vi "Test - Draw Teapot.vi"() -> ()   [LabVIEW 2022 SP3, in "Raster.lvlib"] (continued)
"UV"={"u"=0.0, "v"=0.0}, "Colour"=12517256}, "Vertex 2"={"Position"={"x"=671.18396, "y"=239.12437, "z"=0.9894685}, "UV"={"u"=0.0, "v"=0.0}, "Colour"=12517256}, "Vertex 3"={"Position"={"x"=666.5512, "y"=236.05386, "z"=0.9897306}, "UV"={"u"=0.0, "v"=0.0}, "Colour"=12517256}, "Alpha"=0.0, "Alpha Blending Enabled"=FALSE, "Colour"=131841}, {"Vertex 1"={"Position"={"x"=447.1671, "y"=407.3197, "z"=0.98938274}, "UV"={"u"=0.0, "v"=0.0}, "Colour"=12517256}, "Vertex 2"={"Position"={"x"=434.50436, "y"=408.5937, "z"=0.9895617}, "UV"={"u"=0.0, "v"=0.0}, "Colour"=12517256}, "Vertex 3"={"Position"={"x"=437.53577, "y"=407.4392, "z"=0.98967314}, "UV"={"u"=0.0, "v"=0.0}, "Colour"=12517256}, "Alpha"=0.0, "Alpha Blending Enabled"=FALSE, "Colour"=9618536}, {"Vertex 1"={"Position"={"x"=421.20996, "y"=448.31607, "z"=0.98949325}, "UV"={"u"=0.0, "v"=0.0}, "Colour"=12517256}, "Vertex 2"={"Position"={"x"=417.69724, "y"=440.7109, "z"=0.9895852}, "UV"={"u"=0.0, "v"=0.0}, "Colour"=12517256}, "Vertex 3"={"Position"={"x"=413.86533, "y"=441.3613, "z"=0.9895369}, "UV"={"u"=0.0, "v"=0.0}, "Colour"=12517256}, "Alpha"=0.0, "Alpha Blending Enabled"=FALSE, "Colour"=131841}, {"Vertex 1"={"Position"={"x"=400.0, "y"=130.68715, "z"=0.990049}, "UV"={"u"=0.0, "v"=0.0}, "Colour"=12517256}, "Vertex 2"={"Position"={"x"=413.89853, "y"=117.449425, "z"=0.9892527}, "UV"={"u"=0.0, "v"=0.0}, "Colour"=12517256}, "Vertex 3"={"Position"={"x"=420.06744, "y"=118.36189, "z"=0.9893066}, "UV"={"u"=0.0, "v"=0.0}, "Colour"=12517256}, "Alpha"=0.0, "Alpha Blending Enabled"=FALSE, "Colour"=131841}, {"Vertex 1"={"Position"={"x"=400.0, "y"=130.68715, "z"=0.990049}, "UV"={"u"=0.0, "v"=0.0}, "Colour"=12517256}, "Vertex 2"={"Position"={"x"=379.93253, "y"=118.36189, "z"=0.9893066}, "UV"={"u"=0.0, "v"=0.0}, "Colour"=12517256}, "Vertex 3"={"Position"={"x"=386.10147, "y"=117.449425, "z"=0.9892527}, "UV"={"u"=0.0, "v"=0.0}, "Colour"=12517256}, "Alpha"=0.0, "Alpha Blending Enabled"=FALSE, "Colour"=131841}, {"Vertex 1"={"Position"={"x"=437.2447, "y"=124.60762, "z"=0.98967606}, "UV"={"u"=0.0, "v"=0.0}, "Colour"=12517256}, "Vertex 2"={"Position"={"x"=469.5572, "y"=119.82906, "z"=0.98935246}, "UV"={"u"=0.0, "v"=0.0}, "Colour"=12517256}, "Vertex 3"={"Position"={"x"=472.6678, "y"=123.64719, "z"=0.9895792}, "UV"={"u"=0.0, "v"=0.0}, "Colour"=12517256}, "Alpha"=0.0, "Alpha Blending Enabled"=FALSE, "Colour"=131841}, {"Vertex 1"={"Position"={"x"=406.89297, "y"=415.6739, "z"=0.98965406}, "UV"={"u"=0.0, "v"=0.0}, "Colour"=12517256}, "Vertex 2"={"Position"={"x"=409.7829, "y"=413.03857, "z"=0.9894885}, "UV"={"u"=0.0, "v"=0.0}, "Colour"=12517256}, "Vertex 3"={"Position"={"x"=405.04242, "y"=413.28833, "z"=0.9894651}, "UV"={"u"=0.0, "v"=0.0}, "Colour"=12517256}, "Alpha"=0.0, "Alpha Blending Enabled"=FALSE, "Colour"=11792768}, {"Vertex 1"={"Position"={"x"=271.31854, "y"=391.44998, "z"=0.9896373}, "UV"={"u"=0.0, "v"=0.0}, "Colour"=12517256}, "Vertex 2"={"Position"={"x"=282.90906, "y"=394.1647, "z"=0.98967445}, "UV"={"u"=0.0, "v"=0.0}, "Colour"=12517256}, "Vertex 3"={"Position"={"x"=283.20917, "y"=397.61792, "z"=0.98929393}, "UV"={"u"=0.0, "v"=0.0}, "Colour"=12517256}, "Alpha"=0.0, "Alpha Blending Enabled"=FALSE, "Colour"=9091427}, {"Vertex 1"={"Position"={"x"=314.0461, "y"=401.00818, "z"=0.9894933}, "UV"={"u"=0.0, "v"=0.0}, "Colour"=12517256}, "Vertex 2"={"Position"={"x"=297.89752, "y"=399.48126, "z"=0.9893889}, "UV"={"u"=0.0, "v"=0.0}, "Colour"=12517256}, "Vertex 3"={"Position"={"x"=297.17767, "y"=396.39102, "z"=0.98972005}, "UV"={"u"=0.0, "v"=0.0}, "Colour"=12517256}, "Alpha"=0.0, "Alpha Blending Enabled"=FALSE, "Colour"=9091426}, {"Vertex 1"={"Position"={"x"=469.5572, "y"=119.82906, "z"=0.98935246}, "UV"={"u"=0.0, "v"=0.0}, "Colour"=12517256}, "Vertex 2"={"Position"={"x"=437.2447, "y"=124.60762, "z"=0.98967606}, "UV"={"u"=0.0, "v"=0.0}, "Colour"=12517256}, "Vertex 3"={"Position"={"x"=434.23392, "y"=122.73771, "z"=0.98956543}, "UV"={"u"=0.0, "v"=0.0}, "Colour"=12517256}, "Alpha"=0.0, "Alpha Blending Enabled"=FALSE, "Colour"=131841}, {"Vertex 1"={"Position"={"x"=437.53577, "y"=407.4392, "z"=0.98967314}, "UV"={"u"=0.0, "v"=0.0}, "Colour"=12517256}, "Vertex 2"={"Position"={"x"=451.1117, "y"=405.76608, "z"=0.98953724}, "UV"={"u"=0.0, "v"=0.0}, "Colour"=12517256}, "Vertex 3"={"Position"={"x"=447.1671, "y"=407.3197, "z"=0.98938274}, "UV"={"u"=0.0, "v"=0.0}, "Colour"=12517256}, "Alpha"=0.0, "Alpha Blending Enabled"=FALSE, "Colour"=9618536}, {"Vertex 1"={"Position"={"x"=392.3791, "y"=433.84442, "z"=0.9896132}, "UV"={"u"=0.0, "v"=0.0}, "Colour"=12517256}, "Vertex 2"={"Position"={"x"=390.40692, "y"=441.8486, "z"=0.98950064}, "UV"={"u"=0.0, "v"=0.0}, "Colour"=12517256}, "Vertex 3"={"Position"={"x"=395.05292, "y"=442.15393, "z"=0.98947793}, "UV"={"u"=0.0, "v"=0.0}, "Colour"=12517256}, "Alpha"=0.0, "Alpha Blending Enabled"=FALSE, "Colour"=461317}, {"Vertex 1"={"Position"={"x"=648.9251, "y"=288.04398, "z"=0.9894685}, "UV"={"u"=0.0, "v"=0.0}, "Colour"=12517256}, "Vertex 2"={"Position"={"x"=635.5962, "y"=277.87793, "z"=0.989419}, "UV"={"u"=0.0, "v"=0.0}, "Colour"=12517256}, "Vertex 3"={"Position"={"x"=627.5902, "y"=283.8639, "z"=0.98970413}, "UV"={"u"=0.0, "v"=0.0}, "Colour"=12517256}, "Alpha"=0.0, "Alpha Blending Enabled"=FALSE, "Colour"=10211695}, {"Vertex 1"={"Position"={"x"=396.44946, "y"=415.85388, "z"=0.98963785}, "UV"={"u"=0.0, "v"=0.0}, "Colour"=12517256}, "Vertex 2"={"Position"={"x"=394.9576, "y"=413.28833, "z"=0.9894651}, "UV"={"u"=0.0, "v"=0.0}, "Colour"=12517256}, "Vertex 3"={"Position"={"x"=390.2171, "y"=413.03857, "z"=0.9894885}, "UV"={"u"=0.0, "v"=0.0}, "Colour"=12517256}, "Alpha"=0.0, "Alpha Blending Enabled"=FALSE, "Colour"=11792768}, {"Vertex 1"={"Position"={"x"=690.8386, "y"=314.41168, "z"=0.98944694}, "UV"={"u"=0.0, "v"=0.0}, "Colour"=12517256}, "Vertex 2"={"Position"={"x"=695.06805, "y"=334.79984, "z"=0.98953646}, "UV"={"u"=0.0, "v"=0.0}, "Colour"=12517256}, "Vertex 3"={"Position"={"x"=698.27435, "y"=332.08707, "z"=0.9896034}, "UV"={"u"=0.0, "v"=0.0}, "Colour"=12517256}, "Alpha"=0.0, "Alpha Blending Enabled"=FALSE, "Colour"=7444305}, {"Vertex 1"={"Position"={"x"=425.77792, "y"=410.54718, "z"=0.98937297}, "UV"={"u"=0.0, "v"=0.0}, "Colour"=12517256}, "Vertex 2"={"Position"={"x"=418.06192, "y"=412.10922, "z"=0.98957527}, "UV"={"u"=0.0, "v"=0.0}, "Colour"=12517256}, "Vertex 3"={"Position"={"x"=421.46735, "y"=411.46152, "z"=0.9896358}, "UV"={"u"=0.0, "v"=0.0}, "Colour"=12517256}, "Alpha"=0.0, "Alpha Blending Enabled"=FALSE, "Colour"=10409073}, {"Vertex 1"={"Position"={"x"=409.72174, "y"=462.79736, "z"=0.98969}, "UV"={"u"=0.0, "v"=0.0}, "Colour"=12517256}, "Vertex 2"={"Position"={"x"=415.7588, "y"=463.67755, "z"=0.98946714}, "UV"={"u"=0.0, "v"=0.0}, "Colour"=12517256}, "Vertex 3"={"Position"={"x"=410.90912, "y"=464.3185, "z"=0.98942566}, "UV"={"u"=0.0, "v"=0.0}, "Colour"=12517256}, "Alpha"=0.0, "Alpha Blending Enabled"=FALSE, "Colour"=10343280}, {"Vertex 1"={"Position"={"x"=698.27435, "y"=332.08707, "z"=0.9896034}, "UV"={"u"=0.0, "v"=0.0}, "Colour"=12517256}, "Vertex 2"={"Position"={"x"=693.37805, "y"=310.46698, "z"=0.98952615}, "UV"={"u"=0.0, "v"=0.0}, "Colour"=12517256}, "Vertex 3"={"Position"={"x"=690.8386, "y"=314.41168, "z"=0.98944694}, "UV"={"u"=0.0, "v"=0.0}, "Colour"=12517256}, "Alpha"=0.0, "Alpha Blending Enabled"=FALSE, "Colour"=6522183}, {"Vertex 1"={"Position"={"x"=403.92798, "y"=434.0735, "z"=0.9895953}, "UV"={"u"=0.0, "v"=0.0}, "Colour"=12517256}, "Vertex 2"={"Position"={"x"=404.94708, "y"=442.15393, "z"=0.98947793}, "UV"={"u"=0.0, "v"=0.0}, "Colour"=12517256}, "Vertex 3"={"Position"={"x"=409.59305, "y"=441.8486, "z"=0.98950064}, "UV"={"u"=0.0, "v"=0.0}, "Colour"=12517256}, "Alpha"=0.0, "Alpha Blending Enabled"=FALSE, "Colour"=461317}, {"Vertex 1"={"Position"={"x"=427.9001, "y"=453.91602, "z"=0.98951197}, "UV"={"u"=0.0, "v"=0.0}, "Colour"=12517256}, "Vertex 2"={"Position"={"x"=425.17258, "y"=447.3146, "z"=0.98956454}, "UV"={"u"=0.0, "v"=0.0}, "Colour"=12517256}, "Vertex 3"={"Position"={"x"=421.20996, "y"=448.31607, "z"=0.98949325}, "UV"={"u"=0.0, "v"=0.0}, "Colour"=12517256}, "Alpha"=0.0, "Alpha Blending Enabled"=FALSE, "Colour"=988427}, {"Vertex 1"={"Position"={"x"=657.4915, "y"=300.53033, "z"=0.9895282}, "UV"={"u"=0.0, "v"=0.0}, "Colour"=12517256}, "Vertex 2"={"Position"={"x"=662.8395, "y"=314.53314, "z"=0.9895922}, "UV"={"u"=0.0, "v"=0.0}, "Colour"=12517256}, "Vertex 3"={"Position"={"x"=670.3497, "y"=310.34482, "z"=0.9894408}, "UV"={"u"=0.0, "v"=0.0}, "Colour"=12517256}, "Alpha"=0.0, "Alpha Blending Enabled"=FALSE, "Colour"=9354853}, {"Vertex 1"={"Position"={"x"=403.55054, "y"=415.85388, "z"=0.98963785}, "UV"={"u"=0.0, "v"=0.0}, "Colour"=12517256}, "Vertex 2"={"Position"={"x"=405.04242, "y"=413.28833, "z"=0.9894651}, "UV"={"u"=0.0, "v"=0.0}, "Colour"=12517256}, "Vertex 3"={"Position"={"x"=400.0, "y"=413.3747, "z"=0.9894571}, "UV"={"u"=0.0, "v"=0.0}, "Colour"=12517256}, "Alpha"=0.0, "Alpha Blending Enabled"=FALSE, "Colour"=11924353}, {"Vertex 1"={"Position"={"x"=673.70026, "y"=326.4925, "z"=0.98952615}, "UV"={"u"=0.0, "v"=0.0}, "Colour"=12517256}, "Vertex 2"={"Position"={"x"=670.3497, "y"=310.34482, "z"=0.9894408}, "UV"={"u"=0.0, "v"=0.0}, "Colour"=12517256}, "Vertex 3"={"Position"={"x"=662.8395, "y"=314.53314, "z"=0.9895922}, "UV"={"u"=0.0, "v"=0.0}, "Colour"=12517256}, "Alpha"=0.0, "Alpha Blending Enabled"=FALSE, "Colour"=8630110}, {"Vertex 1"={"Position"={"x"=393.28003, "y"=463.19003, "z"=0.98966503}, "UV"={"u"=0.0, "v"=0.0}, "Colour"=12517256}, "Vertex 2"={"Position"={"x"=389.09088, "y"=464.3185, "z"=0.98942566}, "UV"={"u"=0.0, "v"=0.0}, "Colour"=12517256}, "Vertex 3"={"Position"={"x"=384.2412, "y"=463.67755, "z"=0.98946714}, "UV"={"u"=0.0, "v"=0.0}, "Colour"=12517256}, "Alpha"=0.0, "Alpha Blending Enabled"=FALSE, "Colour"=10343280}, {"Vertex 1"={"Position"={"x"=383.36658, "y"=449.1381, "z"=0.9894347}, "UV"={"u"=0.0, "v"=0.0}, "Colour"=12517256}, "Vertex 2"={"Position"={"x"=386.13464, "y"=441.3613, "z"=0.9895369}, "UV"={"u"=0.0, "v"=0.0}, "Colour"=12517256}, "Vertex 3"={"Position"={"x"=382.30276, "y"=440.7109, "z"=0.9895852}, "UV"={"u"=0.0, "v"=0.0}, "Colour"=12517256}, "Alpha"=0.0, "Alpha Blending Enabled"=FALSE, "Colour"=131841}, {"Vertex 1"={"Position"={"x"=400.0, "y"=415.91602, "z"=0.9896323}, "UV"={"u"=0.0, "v"=0.0}, "Colour"=12517256}, "Vertex 2"={"Position"={"x"=400.0, "y"=413.3747, "z"=0.9894571}, "UV"={"u"=0.0, "v"=0.0}, "Colour"=12517256}, "Vertex 3"={"Position"={"x"=394.9576, "y"=413.28833, "z"=0.9894651}, "UV"={"u"=0.0, "v"=0.0}, "Colour"=12517256}, "Alpha"=0.0, "Alpha Blending Enabled"=FALSE, "Colour"=11924353}, {"Vertex 1"={"Position"={"x"=423.5128, "y"=460.18484, "z"=0.98943293}, "UV"={"u"=0.0, "v"=0.0}, "Colour"=12517256}, "Vertex 2"={"Position"={"x"=420.0997, "y"=462.82288, "z"=0.98952234}, "UV"={"u"=0.0, "v"=0.0}, "Colour"=12517256}, "Vertex 3"={"Position"={"x"=423.8626, "y"=461.78098, "z"=0.98958975}, "UV"={"u"=0.0, "v"=0.0}, "Colour"=12517256}, "Alpha"=0.0, "Alpha Blending Enabled"=FALSE, "Colour"=11133561}, {"Vertex 1"={"Position"={"x"=396.07202, "y"=434.0735, "z"=0.9895953}, "UV"={"u"=0.0, "v"=0.0}, "Colour"=12517256}, "Vertex 2"={"Position"={"x"=395.05292, "y"=442.15393, "z"=0.98947793}, "UV"={"u"=0.0, "v"=0.0}, "Colour"=12517256}, "Vertex 3"={"Position"={"x"=400.0, "y"=442.25943, "z"=0.98947006}, "UV"={"u"=0.0, "v"=0.0}, "Colour"=12517256}, "Alpha"=0.0, "Alpha Blending Enabled"=FALSE, "Colour"=658951}, {"Vertex 1"={"Position"={"x"=400.0, "y"=434.1526, "z"=0.9895892}, "UV"={"u"=0.0, "v"=0.0}, "Colour"=12517256}, "Vertex 2"={"Position"={"x"=400.0, "y"=442.25943, "z"=0.98947006}, "UV"={"u"=0.0, "v"=0.0}, "Colour"=12517256}, "Vertex 3"={"Position"={"x"=404.94708, "y"=442.15393, "z"=0.98947793}, "UV"={"u"=0.0, "v"=0.0}, "Colour"=12517256}, "Alpha"=0.0, "Alpha Blending Enabled"=FALSE, "Colour"=658951}, {"Vertex 1"={"Position"={"x"=423.8626, "y"=461.78098, "z"=0.98958975}, "UV"={"u"=0.0, "v"=0.0}, "Colour"=12517256}, "Vertex 2"={"Position"={"x"=427.8845, "y"=458.98697, "z"=0.9895123}, "UV"={"u"=0.0, "v"=0.0}, "Colour"=12517256}, "Vertex 3"={"Position"={"x"=423.5128, "y"=460.18484, "z"=0.98943293}, "UV"={"u"=0.0, "v"=0.0}, "Colour"=12517256}, "Alpha"=0.0, "Alpha Blending Enabled"=FALSE, "Colour"=11133561}, {"Vertex 1"={"Position"={"x"=537.5546, "y"=128.3227, "z"=0.989609}, "UV"={"u"=0.0, "v"=0.0}, "Colour"=12517256}, "Vertex 2"={"Position"={"x"=521.88995, "y"=127.45417, "z"=0.9896591}, "UV"={"u"=0.0, "v"=0.0}, "Colour"=12517256}, "Vertex 3"={"Position"={"x"=521.76056, "y"=120.85737, "z"=0.98926175}, "UV"={"u"=0.0, "v"=0.0}, "Colour"=12517256}, "Alpha"=0.0, "Alpha Blending Enabled"=FALSE, "Colour"=131841}, {"Vertex 1"={"Position"={"x"=517.09094, "y"=394.1647, "z"=0.98967445}, "UV"={"u"=0.0, "v"=0.0}, "Colour"=12517256}, "Vertex 2"={"Position"={"x"=528.68146, "y"=391.44998, "z"=0.9896373}, "UV"={"u"=0.0, "v"=0.0}, "Colour"=12517256}, "Vertex 3"={"Position"={"x"=528.8192, "y"=395.14902, "z"=0.98921615}, "UV"={"u"=0.0, "v"=0.0}, "Colour"=12517256}, "Alpha"=0.0, "Alpha Blending Enabled"=FALSE, "Colour"=9091427}, {"Vertex 1"={"Position"={"x"=348.88834, "y"=405.76608, "z"=0.98953724}, "UV"={"u"=0.0, "v"=0.0}, "Colour"=12517256}, "Vertex 2"={"Position"={"x"=333.56543, "y"=404.58322, "z"=0.98938376}, "UV"={"u"=0.0, "v"=0.0}, "Colour"=12517256}, "Vertex 3"={"Position"={"x"=330.52844, "y"=402.4644, "z"=0.9895999}, "UV"={"u"=0.0, "v"=0.0}, "Colour"=12517256}, "Alpha"=0.0, "Alpha Blending Enabled"=FALSE, "Colour"=9289061}, {"Vertex 1"={"Position"={"x"=400.0, "y"=130.68715, "z"=0.990049}, "UV"={"u"=0.0, "v"=0.0}, "Colour"=12517256}, "Vertex 2"={"Position"={"x"=407.17038, "y"=116.87585, "z"=0.9892187}, "UV"={"u"=0.0, "v"=0.0}, "Colour"=12517256}, "Vertex 3"={"Position"={"x"=413.89853, "y"=117.449425, "z"=0.9892527}, "UV"={"u"=0.0, "v"=0.0}, "Colour"=12517256}, "Alpha"=0.0, "Alpha Blending Enabled"=FALSE, "Colour"=131841}, {"Vertex 1"={"Position"={"x"=400.0, "y"=130.68715, "z"=0.990049}, "UV"={"u"=0.0, "v"=0.0}, "Colour"=12517256}, "Vertex 2"={"Position"={"x"=386.10147, "y"=117.449425, "z"=0.9892527}, "UV"={"u"=0.0, "v"=0.0}, "Colour"=12517256}, "Vertex 3"={"Position"={"x"=392.82962, "y"=116.87585, "z"=0.9892187}, "UV"={"u"=0.0, "v"=0.0}, "Colour"=12517256}, "Alpha"=0.0, "Alpha Blending Enabled"=FALSE, "Colour"=131841}, {"Vertex 1"={"Position"={"x"=382.30276, "y"=440.7109, "z"=0.9895852}, "UV"={"u"=0.0, "v"=0.0}, "Colour"=12517256}, "Vertex 2"={"Position"={"x"=378.79004, "y"=448.31607, "z"=0.98949325}, "UV"={"u"=0.0, "v"=0.0}, "Colour"=12517256}, "Vertex 3"={"Position"={"x"=383.36658, "y"=449.1381, "z"=0.9894347}, "UV"={"u"=0.0, "v"=0.0}, "Colour"=12517256}, "Alpha"=0.0, "Alpha Blending Enabled"=FALSE, "Colour"=131841}, {"Vertex 1"={"Position"={"x"=683.931, "y"=340.25684, "z"=0.98953646}, "UV"={"u"=0.0, "v"=0.0}, "Colour"=12517256}, "Vertex 2"={"Position"={"x"=680.5069, "y"=322.8259, "z"=0.98944694}, "UV"={"u"=0.0, "v"=0.0}, "Colour"=12517256}, "Vertex 3"={"Position"={"x"=673.70026, "y"=326.4925, "z"=0.98952615}, "UV"={"u"=0.0, "v"=0.0}, "Colour"=12517256}, "Alpha"=0.0, "Alpha Blending Enabled"=FALSE, "Colour"=10540658}, {"Vertex 1"={"Position"={"x"=374.82742, "y"=447.3146, "z"=0.98956454}, "UV"={"u"=0.0, "v"=0.0}, "Colour"=12517256}, "Vertex 2"={"Position"={"x"=372.0999, "y"=453.91602, "z"=0.98951197}, "UV"={"u"=0.0, "v"=0.0}, "Colour"=12517256}, "Vertex 3"={"Position"={"x"=376.47418, "y"=455.0764, "z"=0.9894326}, "UV"={"u"=0.0, "v"=0.0}, "Colour"=12517256}, "Alpha"=0.0, "Alpha Blending Enabled"=FALSE, "Colour"=988427}, {"Vertex 1"={"Position"={"x"=626.93384, "y"=205.09799, "z"=0.989385}, "UV"={"u"=0.0, "v"=0.0}, "Colour"=12517256}, "Vertex 2"={"Position"={"x"=653.6545, "y"=220.1329, "z"=0.989419}, "UV"={"u"=0.0, "v"=0.0}, "Colour"=12517256}, "Vertex 3"={"Position"={"x"=648.53705, "y"=216.88268, "z"=0.98970413}, "UV"={"u"=0.0, "v"=0.0}, "Colour"=12517256}, "Alpha"=0.0, "Alpha Blending Enabled"=FALSE, "Colour"=131841}, {"Vertex 1"={"Position"={"x"=680.5069, "y"=322.8259, "z"=0.98944694}, "UV"={"u"=0.0, "v"=0.0}, "Colour"=12517256}, "Vertex 2"={"Position"={"x"=683.931, "y"=340.25684, "z"=0.98953646}, "UV"={"u"=0.0, "v"=0.0}, "Colour"=12517256}, "Vertex 3"={"Position"={"x"=690.1191, "y"=337.60867, "z"=0.98951393}, "UV"={"u"=0.0, "v"=0.0}, "Colour"=12517256}, "Alpha"=0.0, "Alpha Blending Enabled"=FALSE, "Colour"=10804598}, {"Vertex 1"={"Position"={"x"=376.47418, "y"=455.0764, "z"=0.9894326}, "UV"={"u"=0.0, "v"=0.0}, "Colour"=12517256}, "Vertex 2"={"Position"={"x"=378.79004, "y"=448.31607, "z"=0.98949325}, "UV"={"u"=0.0, "v"=0.0}, "Colour"=12517256}, "Vertex 3"={"Position"={"x"=374.82742, "y"=447.3146, "z"=0.98956454}, "UV"={"u"=0.0, "v"=0.0}, "Colour"=12517256}, "Alpha"=0.0, "Alpha Blending Enabled"=FALSE, "Colour"=988427}, {"Vertex 1"={"Position"={"x"=406.71997, "y"=463.19003, "z"=0.98966503}, "UV"={"u"=0.0, "v"=0.0}, "Colour"=12517256}, "Vertex 2"={"Position"={"x"=410.90912, "y"=464.3185, "z"=0.98942566}, "UV"={"u"=0.0, "v"=0.0}, "Colour"=12517256}, "Vertex 3"={"Position"={"x"=405.62814, "y"=464.7204, "z"=0.9893997}, "UV"={"u"=0.0, "v"=0.0}, "Colour"=12517256}, "Alpha"=0.0, "Alpha Blending Enabled"=FALSE, "Colour"=10409073}, {"Vertex 1"={"Position"={"x"=635.5962, "y"=277.87793, "z"=0.989419}, "UV"={"u"=0.0, "v"=0.0}, "Colour"=12517256}, "Vertex 2"={"Position"={"x"=615.98, "y"=270.86078, "z"=0.989385}, "UV"={"u"=0.0, "v"=0.0}, "Colour"=12517256}, "Vertex 3"={"Position"={"x"=608.8621, "y"=277.8157, "z"=0.9896861}, "UV"={"u"=0.0, "v"=0.0}, "Colour"=12517256}, "Alpha"=0.0, "Alpha Blending Enabled"=FALSE, "Colour"=11265402}, {"Vertex 1"={"Position"={"x"=365.49564, "y"=408.5937, "z"=0.9895617}, "UV"={"u"=0.0, "v"=0.0}, "Colour"=12517256}, "Vertex 2"={"Position"={"x"=352.83286, "y"=407.3197, "z"=0.98938274}, "UV"={"u"=0.0, "v"=0.0}, "Colour"=12517256}, "Vertex 3"={"Position"={"x"=348.88834, "y"=405.76608, "z"=0.98953724}, "UV"={"u"=0.0, "v"=0.0}, "Colour"=12517256}, "Alpha"=0.0, "Alpha Blending Enabled"=FALSE, "Colour"=9618536}, {"Vertex 1"={"Position"={"x"=314.0461, "y"=401.00818, "z"=0.9894933}, "UV"={"u"=0.0, "v"=0.0}, "Colour"=12517256}, "Vertex 2"={"Position"={"x"=330.52844, "y"=402.4644, "z"=0.9895999}, "UV"={"u"=0.0, "v"=0.0}, "Colour"=12517256}, "Vertex 3"={"Position"={"x"=333.56543, "y"=404.58322, "z"=0.98938376}, "UV"={"u"=0.0, "v"=0.0}, "Colour"=12517256}, "Alpha"=0.0, "Alpha Blending Enabled"=FALSE, "Colour"=9289061}, {"Vertex 1"={"Position"={"x"=400.0, "y"=130.68715, "z"=0.990049}, "UV"={"u"=0.0, "v"=0.0}, "Colour"=12517256}, "Vertex 2"={"Position"={"x"=400.0, "y"=116.67725, "z"=0.989207}, "UV"={"u"=0.0, "v"=0.0}, "Colour"=12517256}, "Vertex 3"={"Position"={"x"=407.17038, "y"=116.87585, "z"=0.9892187}, "UV"={"u"=0.0, "v"=0.0}, "Colour"=12517256}, "Alpha"=0.0, "Alpha Blending Enabled"=FALSE, "Colour"=131841}, {"Vertex 1"={"Position"={"x"=400.0, "y"=130.68715, "z"=0.990049}, "UV"={"u"=0.0, "v"=0.0}, "Colour"=12517256}, "Vertex 2"={"Position"={"x"=392.82962, "y"=116.87585, "z"=0.9892187}, "UV"={"u"=0.0, "v"=0.0}, "Colour"=12517256}, "Vertex 3"={"Position"={"x"=400.0, "y"=116.67725, "z"=0.989207}, "UV"={"u"=0.0, "v"=0.0}, "Colour"=12517256}, "Alpha"=0.0, "Alpha Blending Enabled"=FALSE, "Colour"=131841}, {"Vertex 1"={"Position"={"x"=396.5364, "y"=463.4357, "z"=0.9896494}, "UV"={"u"=0.0, "v"=0.0}, "Colour"=12517256}, "Vertex 2"={"Position"={"x"=394.37186, "y"=464.7204, "z"=0.9893997}, "UV"={"u"=0.0, "v"=0.0}, "Colour"=12517256}, "Vertex 3"={"Position"={"x"=389.09088, "y"=464.3185, "z"=0.98942566}, "UV"={"u"=0.0, "v"=0.0}, "Colour"=12517256}, "Alpha"=0.0, "Alpha Blending Enabled"=FALSE, "Colour"=10409073}, {"Vertex 1"={"Position"={"x"=688.6595, "y"=283.87192, "z"=0.9895922}, "UV"={"u"=0.0, "v"=0.0}, "Colour"=12517256}, "Vertex 2"={"Position"={"x"=682.01483, "y"=260.7837, "z"=0.9895282}, "UV"={"u"=0.0, "v"=0.0}, "Colour"=12517256}, "Vertex 3"={"Position"={"x"=683.1556, "y"=265.8486, "z"=0.9893541}, "UV"={"u"=0.0, "v"=0.0}, "Colour"=12517256}, "Alpha"=0.0, "Alpha Blending Enabled"=FALSE, "Colour"=2305817}, {"Vertex 1"={"Position"={"x"=374.2221, "y"=410.54718, "z"=0.98937297}, "UV"={"u"=0.0, "v"=0.0}, "Colour"=12517256}, "Vertex 2"={"Position"={"x"=381.9381, "y"=412.10922, "z"=0.98957527}, "UV"={"u"=0.0, "v"=0.0}, "Colour"=12517256}, "Vertex 3"={"Position"={"x"=385.85406, "y"=412.64026, "z"=0.98952574}, "UV"={"u"=0.0, "v"=0.0}, "Colour"=12517256}, "Alpha"=0.0, "Alpha Blending Enabled"=FALSE, "Colour"=10672500}, {"Vertex 1"={"Position"={"x"=416.63342, "y"=449.1381, "z"=0.9894347}, "UV"={"u"=0.0, "v"=0.0}, "Colour"=12517256}, "Vertex 2"={"Position"={"x"=413.86533, "y"=441.3613, "z"=0.9895369}, "UV"={"u"=0.0, "v"=0.0}, "Colour"=12517256}, "Vertex 3"={"Position"={"x"=409.59305, "y"=441.8486, "z"=0.98950064}, "UV"={"u"=0.0, "v"=0.0}, "Colour"=12517256}, "Alpha"=0.0, "Alpha Blending Enabled"=FALSE, "Colour"=263427}, {"Vertex 1"={"Position"={"x"=686.3912, "y"=318.6656, "z"=0.9894203}, "UV"={"u"=0.0, "v"=0.0}, "Colour"=12517256}, "Vertex 2"={"Position"={"x"=690.1191, "y"=337.60867, "z"=0.98951393}, "UV"={"u"=0.0, "v"=0.0}, "Colour"=12517256}, "Vertex 3"={"Position"={"x"=695.06805, "y"=334.79984, "z"=0.98953646}, "UV"={"u"=0.0, "v"=0.0}, "Colour"=12517256}, "Alpha"=0.0, "Alpha Blending Enabled"=FALSE, "Colour"=9750122}, {"Vertex 1"={"Position"={"x"=421.46735, "y"=411.46152, "z"=0.9896358}, "UV"={"u"=0.0, "v"=0.0}, "Colour"=12517256}, "Vertex 2"={"Position"={"x"=430.5626, "y"=409.63797, "z"=0.98946077}, "UV"={"u"=0.0, "v"=0.0}, "Colour"=12517256}, "Vertex 3"={"Position"={"x"=425.77792, "y"=410.54718, "z"=0.98937297}, "UV"={"u"=0.0, "v"=0.0}, "Colour"=12517256}, "Alpha"=0.0, "Alpha Blending Enabled"=FALSE, "Colour"=10409073}, {"Vertex 1"={"Position"={"x"=379.9003, "y"=462.82288, "z"=0.98952234}, "UV"={"u"=0.0, "v"=0.0}, "Colour"=12517256}, "Vertex 2"={"Position"={"x"=376.4872, "y"=460.18484, "z"=0.98943293}, "UV"={"u"=0.0, "v"=0.0}, "Colour"=12517256}, "Vertex 3"={"Position"={"x"=372.1155, "y"=458.98697, "z"=0.9895123}, "UV"={"u"=0.0, "v"=0.0}, "Colour"=12517256}, "Alpha"=0.0, "Alpha Blending Enabled"=FALSE, "Colour"=11133561}, {"Vertex 1"={"Position"={"x"=263.53796, "y"=388.02435, "z"=0.98961246}, "UV"={"u"=0.0, "v"=0.0}, "Colour"=12517256}, "Vertex 2"={"Position"={"x"=271.31854, "y"=391.44998, "z"=0.9896373}, "UV"={"u"=0.0, "v"=0.0}, "Colour"=12517256}, "Vertex 3"={"Position"={"x"=271.1808, "y"=395.14902, "z"=0.98921615}, "UV"={"u"=0.0, "v"=0.0}, "Colour"=12517256}, "Alpha"=0.0, "Alpha Blending Enabled"=FALSE, "Colour"=8893792}, {"Vertex 1"={"Position"={"x"=413.86533, "y"=441.3613, "z"=0.9895369}, "UV"={"u"=0.0, "v"=0.0}, "Colour"=12517256}, "Vertex 2"={"Position"={"x"=416.63342, "y"=449.1381, "z"=0.9894347}, "UV"={"u"=0.0, "v"=0.0}, "Colour"=12517256}, "Vertex 3"={"Position"={"x"=421.20996, "y"=448.31607, "z"=0.98949325}, "UV"={"u"=0.0, "v"=0.0}, "Colour"=12517256}, "Alpha"=0.0, "Alpha Blending Enabled"=FALSE, "Colour"=131841}, {"Vertex 1"={"Position"={"x"=372.0999, "y"=453.91602, "z"=0.98951197}, "UV"={"u"=0.0, "v"=0.0}, "Colour"=12517256}, "Vertex 2"={"Position"={"x"=372.1155, "y"=458.98697, "z"=0.9895123}, "UV"={"u"=0.0, "v"=0.0}, "Colour"=12517256}, "Vertex 3"={"Position"={"x"=376.4872, "y"=460.18484, "z"=0.98943293}, "UV"={"u"=0.0, "v"=0.0}, "Colour"=12517256}, "Alpha"=0.0, "Alpha Blending Enabled"=FALSE, "Colour"=6785610}, {"Vertex 1"={"Position"={"x"=427.8845, "y"=458.98697, "z"=0.9895123}, "UV"={"u"=0.0, "v"=0.0}, "Colour"=12517256}, "Vertex 2"={"Position"={"x"=427.9001, "y"=453.91602, "z"=0.98951197}, "UV"={"u"=0.0, "v"=0.0}, "Colour"=12517256}, "Vertex 3"={"Position"={"x"=423.52582, "y"=455.0764, "z"=0.9894326}, "UV"={"u"=0.0, "v"=0.0}, "Colour"=12517256}, "Alpha"=0.0, "Alpha Blending Enabled"=FALSE, "Colour"=6785610}, {"Vertex 1"={"Position"={"x"=588.6202, "y"=195.32538, "z"=0.9893725}, "UV"={"u"=0.0, "v"=0.0}, "Colour"=12517256}, "Vertex 2"={"Position"={"x"=626.93384, "y"=205.09799, "z"=0.989385}, "UV"={"u"=0.0, "v"=0.0}, "Colour"=12517256}, "Vertex 3"={"Position"={"x"=621.5498, "y"=201.64421, "z"=0.9896861}, "UV"={"u"=0.0, "v"=0.0}, "Colour"=12517256}, "Alpha"=0.0, "Alpha Blending Enabled"=FALSE, "Colour"=131841}, {"Vertex 1"={"Position"={"x"=403.4636, "y"=463.4357, "z"=0.9896494}, "UV"={"u"=0.0, "v"=0.0}, "Colour"=12517256}, "Vertex 2"={"Position"={"x"=405.62814, "y"=464.7204, "z"=0.9893997}, "UV"={"u"=0.0, "v"=0.0}, "Colour"=12517256}, "Vertex 3"={"Position"={"x"=400.0, "y"=464.85934, "z"=0.98939073}, "UV"={"u"=0.0, "v"=0.0}, "Colour"=12517256}, "Alpha"=0.0, "Alpha Blending Enabled"=FALSE, "Colour"=10474866}, {"Vertex 1"={"Position"={"x"=421.20996, "y"=448.31607, "z"=0.98949325}, "UV"={"u"=0.0, "v"=0.0}, "Colour"=12517256}, "Vertex 2"={"Position"={"x"=423.52582, "y"=455.0764, "z"=0.9894326}, "UV"={"u"=0.0, "v"=0.0}, "Colour"=12517256}, "Vertex 3"={"Position"={"x"=427.9001, "y"=453.91602, "z"=0.98951197}, "UV"={"u"=0.0, "v"=0.0}, "Colour"=12517256}, "Alpha"=0.0, "Alpha Blending Enabled"=FALSE, "Colour"=988427}, {"Vertex 1"={"Position"={"x"=615.98, "y"=270.86078, "z"=0.989385}, "UV"={"u"=0.0, "v"=0.0}, "Colour"=12517256}, "Vertex 2"={"Position"={"x"=588.6202, "y"=267.82214, "z"=0.9893725}, "UV"={"u"=0.0, "v"=0.0}, "Colour"=12517256}, "Vertex 3"={"Position"={"x"=583.19836, "y"=275.50385, "z"=0.9896794}, "UV"={"u"=0.0, "v"=0.0}, "Colour"=12517256}, "Alpha"=0.0, "Alpha Blending Enabled"=FALSE, "Colour"=11660927}, {"Vertex 1"={"Position"={"x"=400.0, "y"=463.52048, "z"=0.98964405}, "UV"={"u"=0.0, "v"=0.0}, "Colour"=12517256}, "Vertex 2"={"Position"={"x"=400.0, "y"=464.85934, "z"=0.98939073}, "UV"={"u"=0.0, "v"=0.0}, "Colour"=12517256}, "Vertex 3"={"Position"={"x"=394.37186, "y"=464.7204, "z"=0.9893997}, "UV"={"u"=0.0, "v"=0.0}, "Colour"=12517256}, "Alpha"=0.0, "Alpha Blending Enabled"=FALSE, "Colour"=10474866}, {"Vertex 1"={"Position"={"x"=388.48337, "y"=449.75494, "z"=0.98939085}, "UV"={"u"=0.0, "v"=0.0}, "Colour"=12517256}, "Vertex 2"={"Position"={"x"=390.40692, "y"=441.8486, "z"=0.98950064}, "UV"={"u"=0.0, "v"=0.0}, "Colour"=12517256}, "Vertex 3"={"Position"={"x"=386.13464, "y"=441.3613, "z"=0.9895369}, "UV"={"u"=0.0, "v"=0.0}, "Colour"=12517256}, "Alpha"=0.0, "Alpha Blending Enabled"=FALSE, "Colour"=263427}, {"Vertex 1"={"Position"={"x"=278.11005, "y"=127.45417, "z"=0.9896591}, "UV"={"u"=0.0, "v"=0.0}, "Colour"=12517256}, "Vertex 2"={"Position"={"x"=262.44534, "y"=128.3227, "z"=0.989609}, "UV"={"u"=0.0, "v"=0.0}, "Colour"=12517256}, "Vertex 3"={"Position"={"x"=261.91296, "y"=120.87895, "z"=0.98915625}, "UV"={"u"=0.0, "v"=0.0}, "Colour"=12517256}, "Alpha"=0.0, "Alpha Blending Enabled"=FALSE, "Colour"=131841}, {"Vertex 1"={"Position"={"x"=376.4872, "y"=460.18484, "z"=0.98943293}, "UV"={"u"=0.0, "v"=0.0}, "Colour"=12517256}, "Vertex 2"={"Position"={"x"=379.9003, "y"=462.82288, "z"=0.98952234}, "UV"={"u"=0.0, "v"=0.0}, "Colour"=12517256}, "Vertex 3"={"Position"={"x"=384.2412, "y"=463.67755, "z"=0.98946714}, "UV"={"u"=0.0, "v"=0.0}, "Colour"=12517256}, "Alpha"=0.0, "Alpha Blending Enabled"=FALSE, "Colour"=11594878}, {"Vertex 1"={"Position"={"x"=670.3497, "y"=310.34482, "z"=0.9894408}, "UV"={"u"=0.0, "v"=0.0}, "Colour"=12517256}, "Vertex 2"={"Position"={"x"=673.70026, "y"=326.4925, "z"=0.98952615}, "UV"={"u"=0.0, "v"=0.0}, "Colour"=12517256}, "Vertex 3"={"Position"={"x"=680.5069, "y"=322.8259, "z"=0.98944694}, "UV"={"u"=0.0, "v"=0.0}, "Colour"=12517256}, "Alpha"=0.0, "Alpha Blending Enabled"=FALSE, "Colour"=10606707}, {"Vertex 1"={"Position"={"x"=528.68146, "y"=391.44998, "z"=0.9896373}, "UV"={"u"=0.0, "v"=0.0}, "Colour"=12517256}, "Vertex 2"={"Position"={"x"=536.46204, "y"=388.02435, "z"=0.98961246}, "UV"={"u"=0.0, "v"=0.0}, "Colour"=12517256}, "Vertex 3"={"Position"={"x"=536.943, "y"=391.80936, "z"=0.98916364}, "UV"={"u"=0.0, "v"=0.0}, "Colour"=12517256}, "Alpha"=0.0, "Alpha Blending Enabled"=FALSE, "Colour"=8893792}, {"Vertex 1"={"Position"={"x"=381.9381, "y"=412.10922, "z"=0.98957527}, "UV"={"u"=0.0, "v"=0.0}, "Colour"=12517256}, "Vertex 2"={"Position"={"x"=374.2221, "y"=410.54718, "z"=0.98937297}, "UV"={"u"=0.0, "v"=0.0}, "Colour"=12517256}, "Vertex 3"={"Position"={"x"=369.4374, "y"=409.63797, "z"=0.98946077}, "UV"={"u"=0.0, "v"=0.0}, "Colour"=12517256}, "Alpha"=0.0, "Alpha Blending Enabled"=FALSE, "Colour"=10409073}, {"Vertex 1"={"Position"={"x"=352.83286, "y"=407.3197, "z"=0.98938274}, "UV"={"u"=0.0, "v"=0.0}, "Colour"=12517256}, "Vertex 2"={"Position"={"x"=365.49564, "y"=408.5937, "z"=0.9895617}, "UV"={"u"=0.0, "v"=0.0}, "Colour"=12517256}, "Vertex 3"={"Position"={"x"=369.4374, "y"=409.63797, "z"=0.98946077}, "UV"={"u"=0.0, "v"=0.0}, "Colour"=12517256}, "Alpha"=0.0, "Alpha Blending Enabled"=FALSE, "Colour"=9816171}, {"Vertex 1"={"Position"={"x"=695.06805, "y"=334.79984, "z"=0.98953646}, "UV"={"u"=0.0, "v"=0.0}, "Colour"=12517256}, "Vertex 2"={"Position"={"x"=690.8386, "y"=314.41168, "z"=0.98944694}, "UV"={"u"=0.0, "v"=0.0}, "Colour"=12517256}, "Vertex 3"={"Position"={"x"=686.3912, "y"=318.6656, "z"=0.9894203}, "UV"={"u"=0.0, "v"=0.0}, "Colour"=12517256}, "Alpha"=0.0, "Alpha Blending Enabled"=FALSE, "Colour"=9223268}, {"Vertex 1"={"Position"={"x"=516.79083, "y"=397.61792, "z"=0.98929393}, "UV"={"u"=0.0, "v"=0.0}, "Colour"=12517256}, "Vertex 2"={"Position"={"x"=502.10248, "y"=399.48126, "z"=0.9893889}, "UV"={"u"=0.0, "v"=0.0}, "Colour"=12517256}, "Vertex 3"={"Position"={"x"=502.8223, "y"=396.39102, "z"=0.98972005}, "UV"={"u"=0.0, "v"=0.0}, "Colour"=12517256}, "Alpha"=0.0, "Alpha Blending Enabled"=FALSE, "Colour"=9091427}, {"Vertex 1"={"Position"={"x"=420.22992, "y"=411.29608, "z"=0.9893006}, "UV"={"u"=0.0, "v"=0.0}, "Colour"=12517256}, "Vertex 2"={"Position"={"x"=414.14594, "y"=412.64026, "z"=0.98952574}, "UV"={"u"=0.0, "v"=0.0}, "Colour"=12517256}, "Vertex 3"={"Position"={"x"=418.06192, "y"=412.10922, "z"=0.98957527}, "UV"={"u"=0.0, "v"=0.0}, "Colour"=12517256}, "Alpha"=0.0, "Alpha Blending Enabled"=FALSE, "Colour"=10672500}, {"Vertex 1"={"Position"={"x"=278.23944, "y"=120.85737, "z"=0.98926175}, "UV"={"u"=0.0, "v"=0.0}, "Colour"=12517256}, "Vertex 2"={"Position"={"x"=299.91116, "y"=121.74838, "z"=0.98940194}, "UV"={"u"=0.0, "v"=0.0}, "Colour"=12517256}, "Vertex 3"={"Position"={"x"=299.14365, "y"=127.179695, "z"=0.98972636}, "UV"={"u"=0.0, "v"=0.0}, "Colour"=12517256}, "Alpha"=0.0, "Alpha Blending Enabled"=FALSE, "Colour"=131841}, {"Vertex 1"={"Position"={"x"=683.1556, "y"=265.8486, "z"=0.9893541}, "UV"={"u"=0.0, "v"=0.0}, "Colour"=12517256}, "Vertex 2"={"Position"={"x"=689.1351, "y"=288.03708, "z"=0.9894408}, "UV"={"u"=0.0, "v"=0.0}, "Colour"=12517256}, "Vertex 3"={"Position"={"x"=688.6595, "y"=283.87192, "z"=0.9895922}, "UV"={"u"=0.0, "v"=0.0}, "Colour"=12517256}, "Alpha"=0.0, "Alpha Blending Enabled"=FALSE, "Colour"=2832671}, {"Vertex 1"={"Position"={"x"=690.1191, "y"=337.60867, "z"=0.98951393}, "UV"={"u"=0.0, "v"=0.0}, "Colour"=12517256}, "Vertex 2"={"Position"={"x"=686.3912, "y"=318.6656, "z"=0.9894203}, "UV"={"u"=0.0, "v"=0.0}, "Colour"=12517256}, "Vertex 3"={"Position"={"x"=680.5069, "y"=322.8259, "z"=0.98944694}, "UV"={"u"=0.0, "v"=0.0}, "Colour"=12517256}, "Alpha"=0.0, "Alpha Blending Enabled"=FALSE, "Colour"=10738549}, {"Vertex 1"={"Position"={"x"=260.69736, "y"=383.67197, "z"=0.98960334}, "UV"={"u"=0.0, "v"=0.0}, "Colour"=12517256}, "Vertex 2"={"Position"={"x"=263.53796, "y"=388.02435, "z"=0.98961246}, "UV"={"u"=0.0, "v"=0.0}, "Colour"=12517256}, "Vertex 3"={"Position"={"x"=263.057, "y"=391.80936, "z"=0.98916364}, "UV"={"u"=0.0, "v"=0.0}, "Colour"=12517256}, "Alpha"=0.0, "Alpha Blending Enabled"=FALSE, "Colour"=6456134}, {"Vertex 1"={"Position"={"x"=335.4686, "y"=116.20814, "z"=0.98913753}, "UV"={"u"=0.0, "v"=0.0}, "Colour"=12517256}, "Vertex 2"={"Position"={"x"=365.76608, "y"=122.73771, "z"=0.98956543}, "UV"={"u"=0.0, "v"=0.0}, "Colour"=12517256}, "Vertex 3"={"Position"={"x"=362.75528, "y"=124.60762, "z"=0.98967606}, "UV"={"u"=0.0, "v"=0.0}, "Colour"=12517256}, "Alpha"=0.0, "Alpha Blending Enabled"=FALSE, "Colour"=131841}, {"Vertex 1"={"Position"={"x"=423.52582, "y"=455.0764, "z"=0.9894326}, "UV"={"u"=0.0, "v"=0.0}, "Colour"=12517256}, "Vertex 2"={"Position"={"x"=423.5128, "y"=460.18484, "z"=0.98943293}, "UV"={"u"=0.0, "v"=0.0}, "Colour"=12517256}, "Vertex 3"={"Position"={"x"=427.8845, "y"=458.98697, "z"=0.9895123}, "UV"={"u"=0.0, "v"=0.0}, "Colour"=12517256}, "Alpha"=0.0, "Alpha Blending Enabled"=FALSE, "Colour"=6785610}, {"Vertex 1"={"Position"={"x"=376.4872, "y"=460.18484, "z"=0.98943293}, "UV"={"u"=0.0, "v"=0.0}, "Colour"=12517256}, "Vertex 2"={"Position"={"x"=376.47418, "y"=455.0764, "z"=0.9894326}, "UV"={"u"=0.0, "v"=0.0}, "Colour"=12517256}, "Vertex 3"={"Position"={"x"=372.0999, "y"=453.91602, "z"=0.98951197}, "UV"={"u"=0.0, "v"=0.0}, "Colour"=12517256}, "Alpha"=0.0, "Alpha Blending Enabled"=FALSE, "Colour"=6785610}, {"Vertex 1"={"Position"={"x"=411.51666, "y"=449.75494, "z"=0.98939085}, "UV"={"u"=0.0, "v"=0.0}, "Colour"=12517256}, "Vertex 2"={"Position"={"x"=409.59305, "y"=441.8486, "z"=0.98950064}, "UV"={"u"=0.0, "v"=0.0}, "Colour"=12517256}, "Vertex 3"={"Position"={"x"=404.94708, "y"=442.15393, "z"=0.98947793}, "UV"={"u"=0.0, "v"=0.0}, "Colour"=12517256}, "Alpha"=0.0, "Alpha Blending Enabled"=FALSE, "Colour"=592902}, {"Vertex 1"={"Position"={"x"=386.13464, "y"=441.3613, "z"=0.9895369}, "UV"={"u"=0.0, "v"=0.0}, "Colour"=12517256}, "Vertex 2"={"Position"={"x"=383.36658, "y"=449.1381, "z"=0.9894347}, "UV"={"u"=0.0, "v"=0.0}, "Colour"=12517256}, "Vertex 3"={"Position"={"x"=388.48337, "y"=449.75494, "z"=0.98939085}, "UV"={"u"=0.0, "v"=0.0}, "Colour"=12517256}, "Alpha"=0.0, "Alpha Blending Enabled"=FALSE, "Colour"=263427}, {"Vertex 1"={"Position"={"x"=536.46204, "y"=388.02435, "z"=0.98961246}, "UV"={"u"=0.0, "v"=0.0}, "Colour"=12517256}, "Vertex 2"={"Position"={"x"=539.3026, "y"=383.67197, "z"=0.98960334}, "UV"={"u"=0.0, "v"=0.0}, "Colour"=12517256}, "Vertex 3"={"Position"={"x"=539.9189, "y"=387.34802, "z"=0.98914444}, "UV"={"u"=0.0, "v"=0.0}, "Colour"=12517256}, "Alpha"=0.0, 
